vi "Calculate window size.vi"(11 "Window bounds":T1) -> (1 "Vertical window size":i16, 3 "Horisontal window size":i16)   [LabVIEW 2020]
uses:
  <vilib>/Utility/miscctls.llb/LVRectTypeDef.ctl
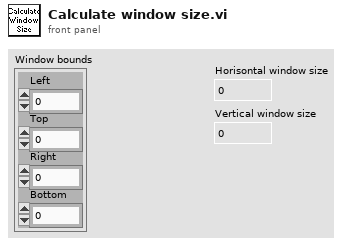
[diagram p1: front panel]
types:
  T1 = typedef "LVRectTypeDef.ctl" = cluster{"Left":i16, "Top":i16, "Right":i16, "Bottom":i16}
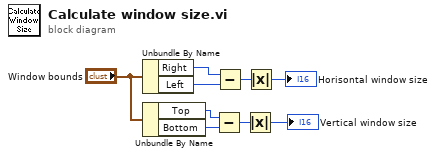
[diagram p0: block diagram]
diagram:
  n1 = Unbundle By Name("Window bounds") -> ("Right"=w9:i16, "Left"=w8:i16)
  n2 = Unbundle By Name("Window bounds") -> ("Top"=w2:i16, "Bottom"=w3:i16)
  n3 = Subtract(x=w2, y=w3) -> (x-y=w4:i16)
  n4 = Subtract(x=w9, y=w8) -> (x-y=w7:i16)
  n5 = Absolute Value(x=w4) -> (abs(x)=→"Vertical window size":i16)
  n6 = Absolute Value(x=w7) -> (abs(x)=→"Horisontal window size":i16)
